vi "NI gRPC Device Server.vi"(8 "error in":errorcluster, 10 "Action":T1) -> (0 "error out":errorcluster)   [LabVIEW 2023]
uses:
  NI gRPC Device Server - Action.ctl
  <vilib>/Utility/sysdir.llb/System Directory Type.ctl
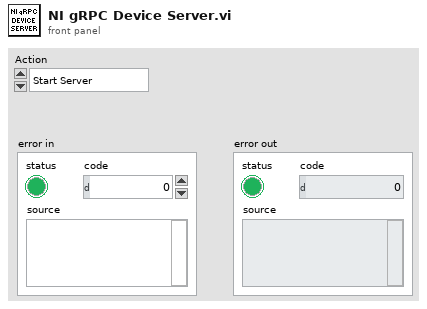
[diagram p1: front panel]
types:
  T1 = typedef "NI gRPC Device Server - Action.ctl" = enum16{"Start Server", "End Server"}
  T2 = typedef "System Directory Type.ctl" = i32
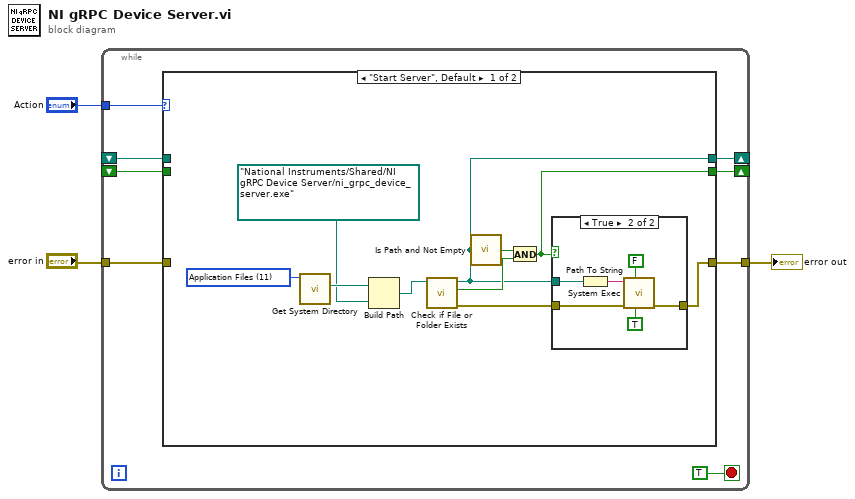
[diagram p0: block diagram]
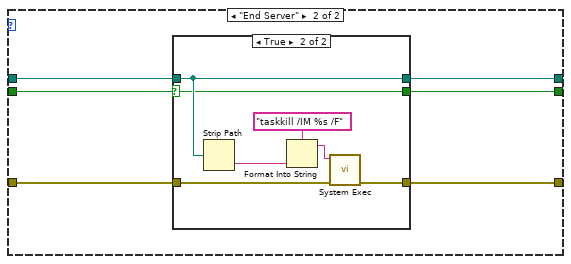
[diagram p3: hidden frame]
diagram:
  n1 = while {
    tunnel: [w11] -> w1
    tunnel: "Action" -> [w10]
    shift-right: [w9] -> _
    shift-left: _ -> [w8]
    tunnel: "error in" -> [w7]
    shift-right: [w5] -> _
    shift-left: _ -> [w4]
    stop <- TRUE stop-if-true
    n2 = case shown="\"Start Server\", Default" w10 {
      tunnel: [w20 w33] -> w11
      tunnel: [w17 w30] -> w9
      tunnel: w8 -> [_ w32]
      tunnel: w7 -> [_ w34]
      tunnel: [w16 w29] -> w5
      tunnel: w4 -> [_ w31]
      frame "Start Server", Default {
        w15 = T2 11 items=["User Home"=0, "User Desktop"=1, "User Documents"=2, "User Application Data"=3, "User Preferences"=4, "User Temporary"=5, "Public Documents"=6, "Public Application Data"=7, "Public Preferences"=8, "Public Cache"=13, "System Core Libraries"=9, "System Installed Libraries"=10, "Application Files"=11, "Boot Volume Root"=12] ("system directory type")
        n3 = call <vilib>:"Get System Directory.vi"("system directory type"=w15) -> ("system directory"=w14:path)  [unwired: 10 in]
        n4 = Build Path(base path=w14, name or relative path=path "National Instruments/Shared/NI gRPC Device Server/ni_grpc_device_server.exe") -> (appended path=w12:path)
        n5 = call <vilib>:"Check if File or Folder Exists.vi"("path"=w12) -> ("error out"=w21:errorcluster, "file or folder exists?"=w18:bool, "dup path"=w17:path)  [unwired: 8 in]
        n6 = call <vilib>:"Is Path and Not Empty.vi"("path"=w17) -> ("Is Path and Not Empty?"=w19:bool)  [unwired: 4 in]
        n7 = And(x=w19, y=w18) -> (x .and. y?=w16:bool)
        n8 = case shown="True" w16 {
          tunnel: w21 -> [w22 w28]
          tunnel: w17 -> [_ w25]
          tunnel: [w22 w23] -> w20
          frame False {
          }
          frame True {
            n9 = Path To String(path=w25) -> (string=w27:string)
            n10 = call <vilib>:"System Exec.vi"("run minimized? (F)"=TRUE, "wait until completion? (T)"=FALSE, "error in (no error)"=w28, "command line"=w27) -> ("error out"=w23:errorcluster)  [unwired: 4 in, 3 out]
          }
        }
      }
      frame "End Server" {
        n11 = case shown="True" w31 {
          selector: w31 -> [w35 w38]
          tunnel: w34 -> [w37 w42]
          tunnel: [w37 w41] -> w33
          tunnel: w32 -> [w36 w39]
          tunnel: [w36 w39] -> w30
          tunnel: [w35 w38] -> w29
          frame False {
          }
          frame True {
            n12 = Strip Path(path=w39) -> (name=w40:string)  [unwired: 1 out]
            n13 = Format Into String(format string="taskkill /IM %s /F", w40) -> (resulting string=w44:string)  [unwired: 2 in, 1 out]
            n14 = call <vilib>:"System Exec.vi"("error in (no error)"=w42, "command line"=w44) -> ("error out"=w41:errorcluster)  [unwired: 6 in, 3 out]
          }
        }
      }
    }
  }
  "error out" <- w1
